vi "New Test Redis Client.vi"(8 "error in (no error)":errorcluster, 9 "timeout (ms)":i32=1000) -> (0 "error out":errorcluster, 1 "receive queue":refnum<queue>, 2 "send queue":refnum<queue>, 3 "Test Redis Client out":refnum<class "Test Redis Client.lvclass">)   [LabVIEW 2019, in "Test Redis Client for LabVIEW.lvlib" / "Test Redis Client.lvclass"]
uses:
  Test Redis Client.lvclass
  Test Redis Client.lvclass/Test Redis Client.ctl
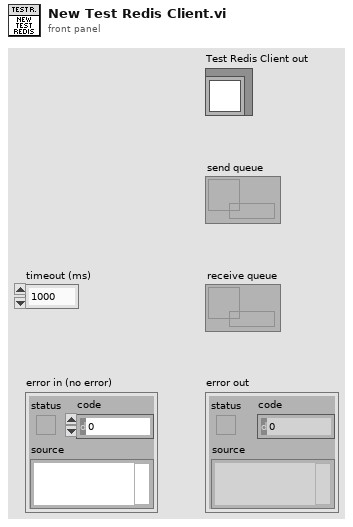
[diagram p1: front panel]
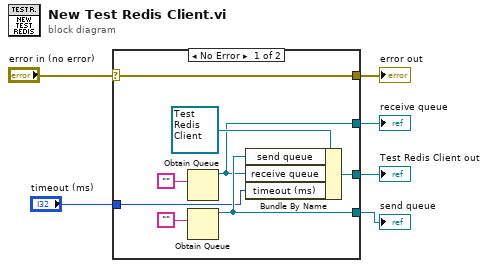
[diagram p0: block diagram]
diagram:
  n1 = case shown="No Error" "error in (no error)" {
    selector: "error in (no error)" -> [w14 w15]
    tunnel: [w14 w15] -> w5
    tunnel: [w8 _] -> w4
    tunnel: [w10 _] -> w3
    tunnel: [w9 _] -> w2
    tunnel: "timeout (ms)" -> [w7 _]
    frame No Error {
      n2 = Obtain Queue(element data type="") -> (queue out=w9:refnum<queue>)  [unwired: 4 in, 2 out]
      n3 = Obtain Queue(element data type="") -> (queue out=w10:refnum<queue>)  [unwired: 4 in, 2 out]
      n4 = Bundle By Name(cluster=refnum<class "Test Redis Client.lvclass"> refnum ("Test Redis Client in"), "send queue"=w10, "receive queue"=w9, "timeout (ms)"=w7) -> (w8:refnum<class "Test Redis Client.lvclass">)
    }
    frame Error {
    }
  }
  "error out" <- w5
  "Test Redis Client out" <- w4
  "send queue" <- w3
  "receive queue" <- w2
